vi "OAT Single Stage Interpolator Decimator Design.vi"(7 "alias free":bool, 9 "A stop [dB]":dbl=72.0 format="%.2f", 10 "bandwidth (auto)":cluster{"passband":dbl, "stopband":dbl} {"stopband" format="%.2f"; "passband" format="%.2f"}, 11 "interpolation/decimation factor":i32=2) -> (0 "error out":errorcluster, 1 "filter":T1={"coefficients"=[], "factor"=1} {"coefficients" format="%.2f"})   [LabVIEW 2017, in "SoundVib_Resampling.lvlib"]
doc: "Design a single stage interpolation/decimation FIR filter."
uses:
  <vilib>/addons/Sound and Vibration/Order Analysis/Resample Order Tracking/SoundVib_Resampling.lvlib
  <vilib>/addons/_NISVFA/_Shared subVIs/Controls/OAT Decimation Filter.ctl
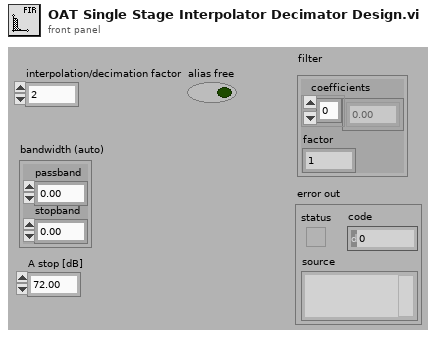
[diagram p1: front panel]
types:
  T1 = typedef "OAT Decimation Filter.ctl" = cluster{"coefficients":dbl[], "factor":i32}
  T2 = cluster{"interpolation/decimation factor":i32, "passband":dbl, "stopband":dbl, "A stop [dB]":dbl}
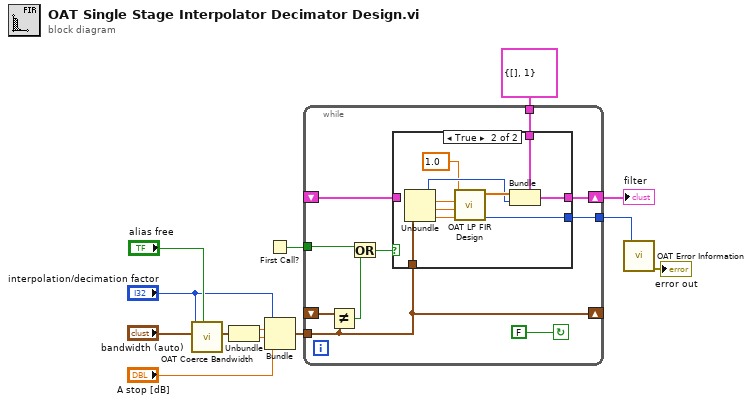
[diagram p0: block diagram]
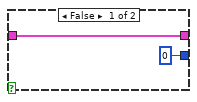
[diagram p2: hidden frame]
diagram:
  n1 = call <vilib>:"OAT Coerce Bandwidth.vi"("alias free"="alias free", "bandwidth (auto)"="bandwidth (auto)", "interpolation/decimation factor"="interpolation/decimation factor") -> ("bandwidth out"=w6:cluster{"passband":dbl, "stopband":dbl})  [unwired: 8 in]
  n2 = Unbundle(w6) -> ("passband"=w5:dbl, "stopband"=w4:dbl)
  n3 = First Call?() -> (First Call?: T/F=w12:bool)
  n4 = Bundle("interpolation/decimation factor"="interpolation/decimation factor", "passband"=w5, "stopband"=w4, "A stop [dB]"="A stop [dB]") -> (w13:T2)  [unwired: 1 in]
  n5 = while {
    shift-right: [w23] -> w11
    shift-left: _ -> [w16]
    shift-right: [w17] -> _
    shift-left: _ -> [w19]
    tunnel: w13 -> [w17]
    tunnel: w12 -> [w18]
    tunnel: T1 {"coefficients"=[], "factor"=1} ("filter") -> [w15]
    tunnel: [w14] -> w2
    stop <- FALSE continue-if-true
    n6 = Not Equal?(x=w19, y=w17) -> (x != y?=w21:bool)
    n7 = Or(x=w18, y=w21) -> (x .or. y?=w20:bool)
    n8 = case shown="True" w20 {
      tunnel: [w25 w34] -> w23
      tunnel: w16 -> [w25 _]
      tunnel: w17 -> [_ w35]
      tunnel: w15 -> [_ w28]
      tunnel: [0 ("error") w26] -> w14
      frame False {
      }
      frame True {
        n9 = Unbundle(w35) -> ("interpolation/decimation factor"=w32:i32, "passband"=w31:dbl, "stopband"=w29:dbl, "A stop [dB]"=w30:dbl)
        n10 = call <vilib>:"OAT LP FIR Design.vi"("A stop [dB]"=w30, "stopband"=w29, "passband"=w31, "fs"=1.0) -> ("error"=w26:i32, "filter coefficients"=w33:dbl[])  [unwired: 6 in]
        n11 = Bundle(cluster=w28, "coefficients"=w33, "factor"=w32) -> (w34:T1)
      }
    }
  }
  "filter" <- w11
  n12 = call <vilib>:"OAT Error Information.vi"("error code"=w2) -> ("error out"=→"error out":errorcluster)  [unwired: 6 in]
